vi "Formula_6.2.vi"(8 "temprature":dbl, 9 "KG":dbl, 10 "KG20":dbl[](array[numeric]), 11 "KTU In":dbl[](array[numeric])) -> (2 "ktu":dbl, 3 "KTU Out":dbl[](array[numeric]))   [LabVIEW 2015]
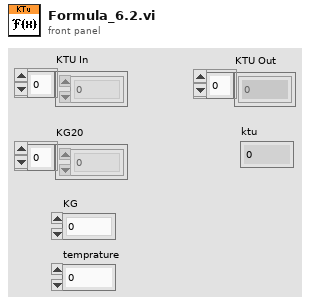
[diagram p1: front panel]
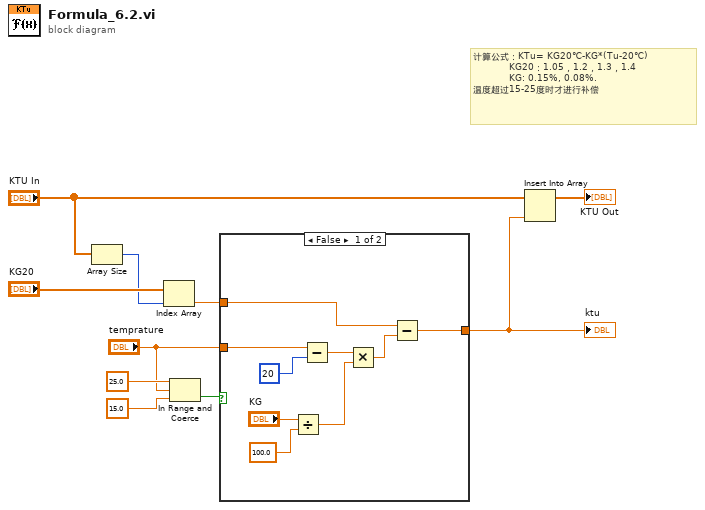
[diagram p0: block diagram]
diagram:
  # "计算公式：KTu= KG20℃-KG*(Tu-20℃)\n            KG20：1.05，1.2，1.3，1.4\n            KG: 0.15%, 0.08%.\n温度超过15-25度时才进行补偿"
  n1 = Array Size(array="KTU In") -> (size(s)=w2:i32)
  n2 = Index Array(array="KG20", index=w2) -> (element=w7:dbl)
  n3 = In Range and Coerce(upper limit=25.0, x="temprature", lower limit=15.0) -> (In Range?=w8:bool)  [unwired: 1 out]
  n4 = case shown="False" w8 {
    tunnel: w7 -> [w12 w20]
    tunnel: [w11 w20] -> w1
    tunnel: "temprature" -> [w13 _]
    frame False {
      n5 = Divide(x="KG", y=100.0) -> (x/y=w15:dbl)
      n6 = Subtract(x=w13, y=20) -> (x-y=w18:dbl)
      n7 = Multiply(x=w18, y=w15) -> (x*y=w17:dbl)
      n8 = Subtract(x=w12, y=w17) -> (x-y=w11:dbl)
    }
    frame True {
    }
  }
  "ktu" <- w1
  n9 = Insert Into Array(array="KTU In", new element=w1) -> (→"KTU Out":dbl[])  [unwired: 1 in]
